vi "Save Project.vi"(0 "project reference":refnum<vi>, 5 "measurement core reference":refnum<vi>, 7 "project path":path, 11 "error in":errorcluster) -> (15 "error out":errorcluster)   [LabVIEW 2021, in "Multiple Converter.lvlib"]
uses:
  Multiple Converter.lvlib
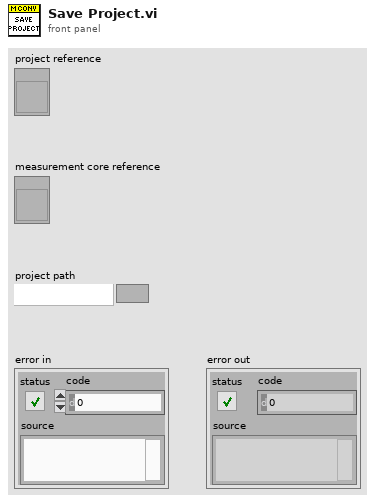
[diagram p1: front panel]
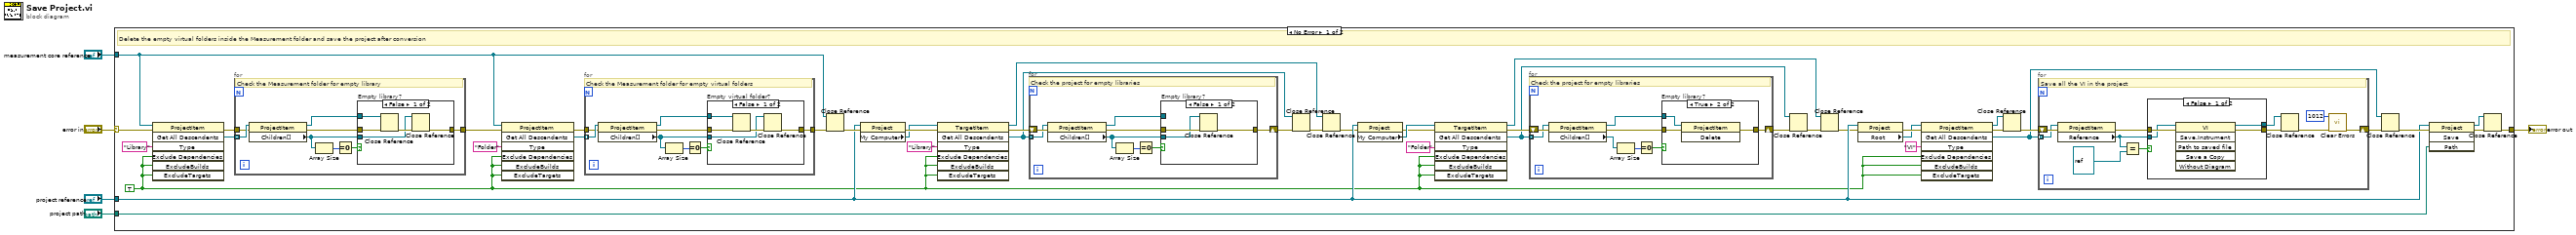
[diagram p0: block diagram]
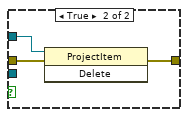
[diagram p2: hidden frame]
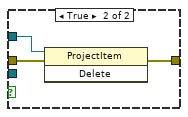
[diagram p4: hidden frame]
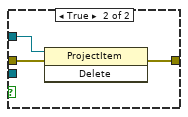
[diagram p5: hidden frame]
diagram:
  n1 = case shown="No Error" "error in" {
    selector: "error in" -> [w14 w125]
    tunnel: [w48 w125] -> w5
    tunnel: "project path" -> [w44 _]
    tunnel: "measurement core reference" -> [w12 _]
    tunnel: "project reference" -> [w23 _]
    frame No Error {
      w6 = TRUE
      # "Delete the empty virtual folders inside the Measurement folder and save the project after conversion"
      n2 = invoke class="ProjectItem" method="Get All Descendents"(reference=w12, error in=w14, "Type"="Library", "Exclude Dependencies"=w6, "ExcludeBuilds"=w6, "ExcludeTargets"=w6) -> (error out=w16:errorcluster, "All Descendents"=w17:refnum<vi>[])  [unwired: 1 in, 5 out]
      n3 = for {
        tunnel: w17 -> [w57] mode=indexing
        tunnel: w16 -> [w56]
        tunnel: [w51] -> w13
        # "Check the Measurement folder for empty library"
        n4 = property class="ProjectItem"(reference=w57, error in=w56) -> (reference out=w52:refnum<vi>, error out=w54:errorcluster, "Children[]"=w50:refnum<vi>[])
        n5 = Array Size(array=w50) -> (size(s)=w55:i32)
        n6 = Equal To 0?(x=w55) -> (x = 0?=w53:bool)
        n7 = case "Empty library?" shown="False" w53 {
          tunnel: w54 -> [w62 w65]
          tunnel: w52 -> [w61 w64]
          tunnel: [w59 w63] -> w51
          tunnel: w50 -> [w58 _]
          frame False {
            n8 = Close Reference(reference=w61, error in (no error)=w62) -> (error out=w60:errorcluster)
            n9 = Close Reference(reference=w58, error in (no error)=w60) -> (error out=w59:errorcluster)
          }
          frame True {
            n10 = invoke class="ProjectItem" method="Delete"(reference=w64, error in=w65) -> (error out=w63:errorcluster)  [unwired: 1 in, 2 out]
          }
        }
      }
      n11 = invoke class="ProjectItem" method="Get All Descendents"(reference=w12, error in=w13, "Type"="Folder", "Exclude Dependencies"=w6, "ExcludeBuilds"=w6, "ExcludeTargets"=w6) -> (error out=w45:errorcluster, "All Descendents"=w34:refnum<vi>[])  [unwired: 1 in, 5 out]
      n12 = for {
        tunnel: w34 -> [w85] mode=indexing
        tunnel: w45 -> [w84]
        tunnel: [w79] -> w28
        # "Check the Measurement folder for empty virtual folders"
        n13 = property class="ProjectItem"(reference=w85, error in=w84) -> (reference out=w80:refnum<vi>, error out=w82:errorcluster, "Children[]"=w78:refnum<vi>[])
        n14 = Array Size(array=w78) -> (size(s)=w83:i32)
        n15 = Equal To 0?(x=w83) -> (x = 0?=w81:bool)
        n16 = case "Empty virtual folder?" shown="False" w81 {
          tunnel: w82 -> [w90 w93]
          tunnel: w80 -> [w89 w92]
          tunnel: [w87 w91] -> w79
          tunnel: w78 -> [w86 _]
          frame False {
            n17 = Close Reference(reference=w89, error in (no error)=w90) -> (error out=w88:errorcluster)
            n18 = Close Reference(reference=w86, error in (no error)=w88) -> (error out=w87:errorcluster)
          }
          frame True {
            n19 = invoke class="ProjectItem" method="Delete"(reference=w92, error in=w93) -> (error out=w91:errorcluster)  [unwired: 1 in, 2 out]
          }
        }
      }
      n20 = Close Reference(reference=w12, error in (no error)=w28) -> (error out=w27:errorcluster)
      n21 = property class="Project"(reference=w23, error in=w27) -> (error out=w38:errorcluster, "My Computer"=w29:refnum<vi>)  [unwired: 1 out]
      n22 = invoke class="TargetItem" method="Get All Descendents"(reference=w29, error in=w38, "Type"="Library", "Exclude Dependencies"=w6, "ExcludeBuilds"=w6, "ExcludeTargets"=w6) -> (reference out=w10:refnum<vi>, error out=w36:errorcluster, "All Descendents"=w32:refnum<vi>[])  [unwired: 1 in, 4 out]
      n23 = for {
        shift-right: [w95] -> w33
        shift-left: w36 -> [w101]
        tunnel: w32 -> [w100] mode=indexing
        # "Check the project for empty libraries"
        n24 = property class="ProjectItem"(reference=w100, error in=w101) -> (reference out=w97:refnum<vi>, error out=w96:errorcluster, "Children[]"=w94:refnum<vi>[])
        n25 = Array Size(array=w94) -> (size(s)=w99:i32)
        n26 = Equal To 0?(x=w99) -> (x = 0?=w98:bool)
        n27 = case "Empty library?" shown="False" w98 {
          tunnel: w96 -> [w104 w107]
          tunnel: w97 -> [_ w106]
          tunnel: [w103 w105] -> w95
          tunnel: w94 -> [w102 _]
          frame False {
            n28 = Close Reference(reference=w102, error in (no error)=w104) -> (error out=w103:errorcluster)
          }
          frame True {
            n29 = invoke class="ProjectItem" method="Delete"(reference=w106, error in=w107) -> (error out=w105:errorcluster)  [unwired: 1 in, 2 out]
          }
        }
      }
      n30 = Close Reference(reference=w32, error in (no error)=w33) -> (error out=w22:errorcluster)
      n31 = Close Reference(reference=w10, error in (no error)=w22) -> (error out=w11:errorcluster)
      n32 = property class="Project"(reference=w23, error in=w11) -> (error out=w24:errorcluster, "My Computer"=w26:refnum<vi>)  [unwired: 1 out]
      n33 = invoke class="TargetItem" method="Get All Descendents"(reference=w26, error in=w24, "Type"="Folder", "Exclude Dependencies"=w6, "ExcludeBuilds"=w6, "ExcludeTargets"=w6) -> (reference out=w8:refnum<vi>, error out=w21:errorcluster, "All Descendents"=w18:refnum<vi>[])  [unwired: 1 in, 4 out]
      n34 = for {
        shift-right: [w66] -> w20
        shift-left: w21 -> [w73]
        tunnel: w18 -> [w72] mode=indexing
        # "Check the project for empty libraries"
        n35 = property class="ProjectItem"(reference=w72, error in=w73) -> (reference out=w68:refnum<vi>, error out=w67:errorcluster, "Children[]"=w70:refnum<vi>[])
        n36 = Array Size(array=w70) -> (size(s)=w71:i32)
        n37 = Equal To 0?(x=w71) -> (x = 0?=w69:bool)
        n38 = case "Empty library?" shown="True" w69 {
          tunnel: w67 -> [w74 w77]
          tunnel: w68 -> [_ w76]
          tunnel: [w74 w75] -> w66
          frame False {
          }
          frame True {
            n39 = invoke class="ProjectItem" method="Delete"(reference=w76, error in=w77) -> (error out=w75:errorcluster)  [unwired: 1 in, 2 out]
          }
        }
      }
      n40 = Close Reference(reference=w18, error in (no error)=w20) -> (error out=w19:errorcluster)
      n41 = Close Reference(reference=w8, error in (no error)=w19) -> (error out=w9:errorcluster)
      n42 = property class="Project"(reference=w23, error in=w9) -> (error out=w43:errorcluster, "Root"=w42:refnum<vi>)  [unwired: 1 out]
      n43 = invoke class="ProjectItem" method="Get All Descendents"(reference=w42, error in=w43, "Type"="VI", "Exclude Dependencies"=w6, "ExcludeBuilds"=w6, "ExcludeTargets"=w6) -> (reference out=w40:refnum<vi>, error out=w41:errorcluster, "All Descendents"=w7:refnum<vi>[])  [unwired: 1 in, 4 out]
      n44 = Close Reference(reference=w40, error in (no error)=w41) -> (error out=w39:errorcluster)
      n45 = for {
        shift-right: [w111] -> w31
        shift-left: w39 -> [w117]
        tunnel: w7 -> [w115] mode=indexing
        # "Save all the VI in the project"
        n46 = property class="ProjectItem"(reference=w115, error in=w117) -> (error out=w116:errorcluster, "Reference"=w112:refnum<vi>)  [unwired: 1 out]
        n47 = Equal?(x=w112, y=refnum<vi> refnum) -> (x = y?=w113:bool)
        n48 = case shown="False" w113 {
          tunnel: [w120 w124] -> w118
          tunnel: w116 -> [w122 w124]
          tunnel: w112 -> [w121 w123]
          tunnel: [w119 w123] -> w108
          frame False {
            n49 = invoke class="VI" method="Save.Instrument"(reference=w121, error in=w122) -> (reference out=w119:refnum<vi>, error out=w120:errorcluster)  [unwired: 4 in, 4 out]
          }
          frame True {
          }
        }
        n50 = Close Reference(reference=w108, error in (no error)=w118) -> (error out=w109:errorcluster)
        n51 = call <vilib>:"Clear Errors.vi"("error in (no error)"=w109, "specific error code to clear (0: all)"=1012) -> ("error out"=w111:errorcluster)  [unwired: 4 in, 1 out]
      }
      n52 = Close Reference(reference=w7, error in (no error)=w31) -> (error out=w30:errorcluster)
      n53 = invoke class="Project" method="Save"(reference=w23, error in=w30, "Path"=w44) -> (reference out=w49:refnum<vi>, error out=w47:errorcluster)  [unwired: 1 in, 2 out]
      n54 = Close Reference(reference=w49, error in (no error)=w47) -> (error out=w48:errorcluster)
    }
    frame Error {
    }
  }
  "error out" <- w5
